vi "Facade.vi"(0 "Data In":T1 caption="数据输入", 2 "Display State In":T4={"method"=enum."None", "current color"=1, "available black position"=[], "available white position"=[], "Interactive Action"=refnum, "row"=0, "column"=0} caption="显示状态输入", 3 "Container State":T7 caption="容器状态") -> (6 "Data Out":T1 caption="数据输出", 7 "Display State Out":T4={"method"=enum."None", "current color"=1, "available black position"=[], "available white position"=[], "Interactive Action"=refnum, "row"=0, "column"=0} caption="显示状态输出", 8 "Action":T3 caption="动作")   [LabVIEW 2011, in "Othello.xctl"]
doc: "查看程序详细说明请访问：http://ruanqizhen.spaces.live.com/blog/cns!5852D4F797C53FB6!3382.entry"
uses:
  Othello.xctl
  Data.ctl
  Control/Pict Ring Chess.ctl
  <vilib>/_xctls/Container State.ctl
  State.ctl
  Control/Method Call.ctl
  Control/Interactive Action.ctl
  <vilib>/_xctls/Action.ctl
  <vilib>/_xctls/XControlSupport.lvlib
panel:
  out "chesses":T1
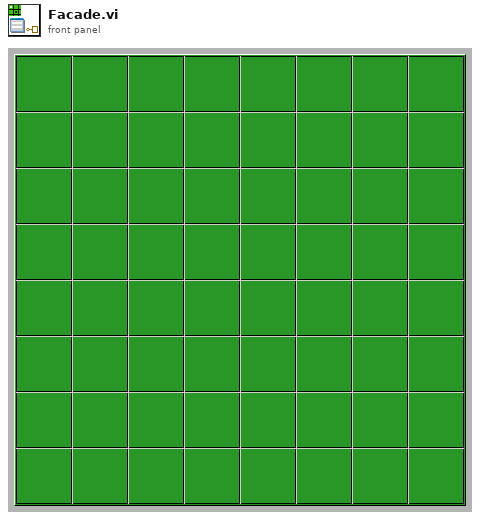
[diagram p1: front panel]
types:
  T1 = typedef "Othello.xctl/Data.ctl" = T2[][]
  T2 = typedef "Othello.xctl/Pict Ring Chess.ctl" = u16
  T3 = typedef "XControlSupport.lvlib/Action.ctl" = cluster{"Data Changed?":bool, "State Changed?":bool, "Action Name":string}
  T4 = typedef "Othello.xctl/State.ctl" = cluster{"method":T5, "current color":T2, "available black position":i32[][], "available white position":i32[][], "Interactive Action":T6, "row":i32, "column":i32}
  T5 = typedef "Othello.xctl/Method Call.ctl" = enum16{"None", "New Game", "Play One"}
  T6 = typedef "Othello.xctl/Interactive Action.ctl" = refnum<user-event>
  T7 = typedef "XControlSupport.lvlib/Container State.ctl" = cluster{"Indicator?":bool, "Run Mode?":bool, " Refnum":refnum<vi>}
  T8 = typedef "LVPoint32TypeDef.ctl" = cluster{"Horizontal":i32, "Vertical":i32}
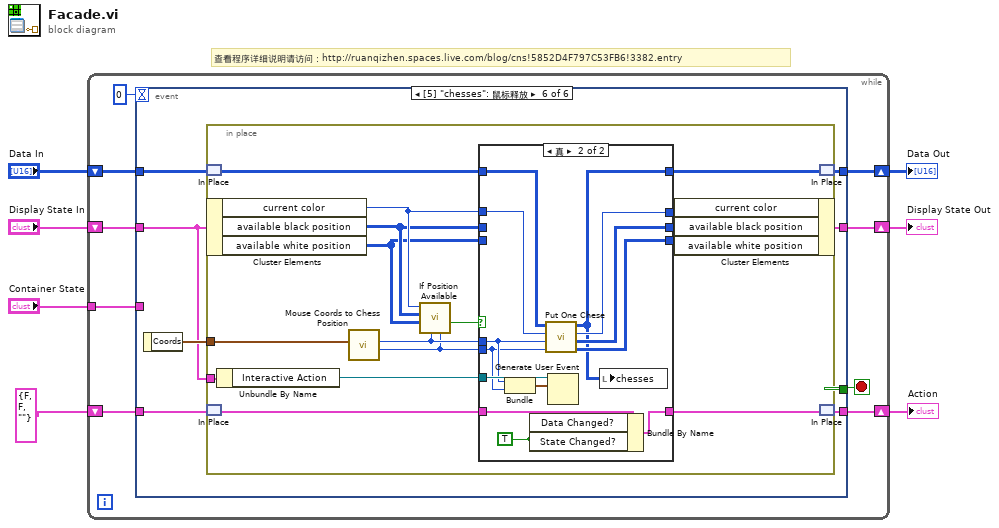
[diagram p0: block diagram]
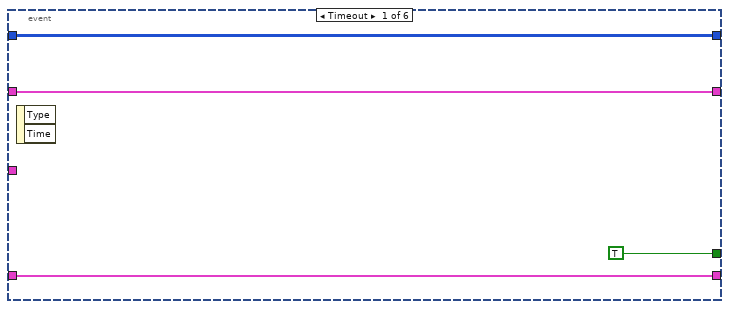
[diagram p2: hidden frame]
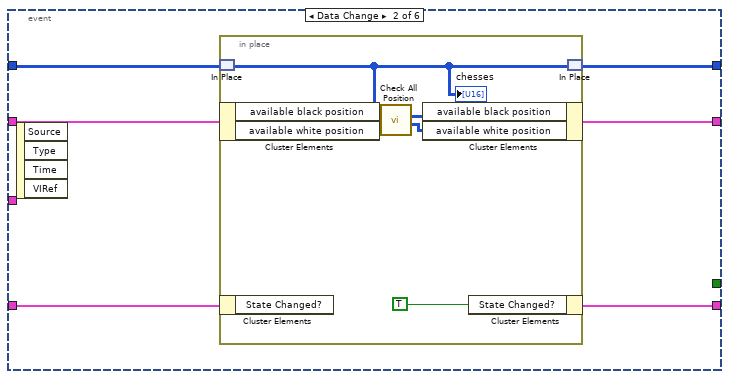
[diagram p3: hidden frame]
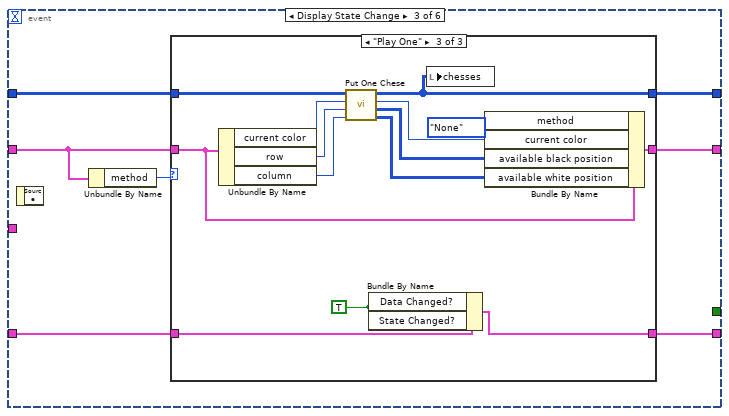
[diagram p4: hidden frame]
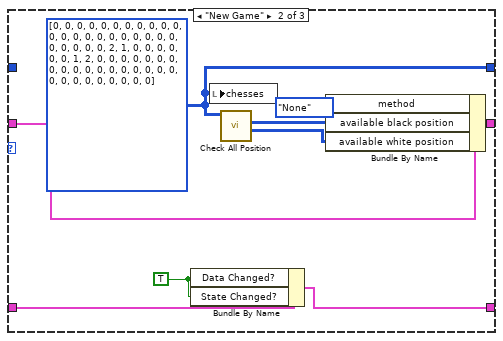
[diagram p6: hidden frame]
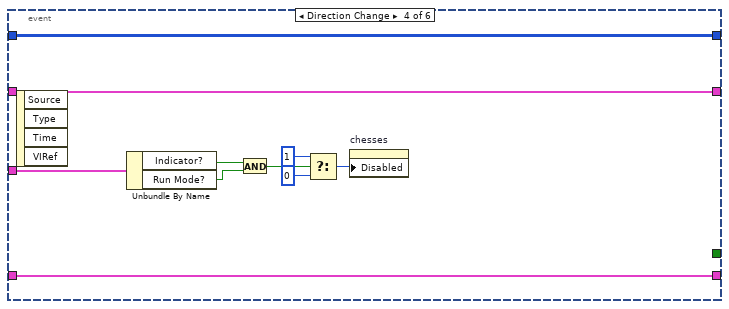
[diagram p7: hidden frame]
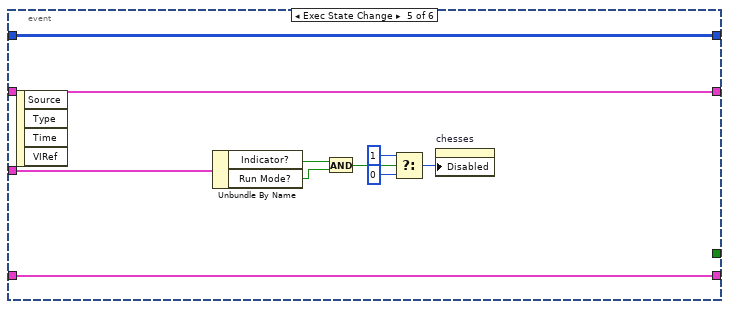
[diagram p8: hidden frame]
diagram:
  # "查看程序详细说明请访问：http://ruanqizhen.spaces.live.com/blog/cns!5852D4F797C53FB6!3382.entry"
  n1 = while {
    shift-right: [w15] -> w4
    shift-left: "Display State In" -> [w16]
    tunnel: "Container State" -> [w12]
    shift-right: [w10] -> w7
    shift-left: "Data In" -> [w11]
    shift-right: [w8] -> w2
    shift-left: T3 {"Data Changed?"=FALSE, "State Changed?"=FALSE, "Action Name"=""} ("Action") -> [w9]
    stop <- w14 stop-if-true
    n2 = event shown="[5] \"chesses\": 鼠标释放" {
      selector: _ -> [_ _ _ _ _ _]
      dyn-events: _ -> [_ _ _ _ _ _]
      timeout: 0 -> [_ _ _ _ _ _]
      tunnel: w16 -> [w18 w25 w33 w72 w83 w86]
      tunnel: [w18 w23 w31 w72 w83 w87] -> w15
      tunnel: [TRUE _ _ _ _ _] -> w14
      tunnel: w12 -> [_ _ _ w73 w74 _]
      tunnel: w11 -> [w17 w22 w36 w71 w82 w89]
      tunnel: [w17 w21 w35 w71 w82 w88] -> w10
      tunnel: [w19 w24 w37 w70 w81 w84] -> w8
      tunnel: w9 -> [w19 w26 w34 w70 w81 w85]
      event Timeout {
        n3 = event-data() -> ()  [unwired: 3 out]
      }
      event Data Change {
        n4 = event-data() -> ()  [unwired: 5 out]
        n5 = in-place {
          n6 = in-place-match #1(w22) -> (w27:T1)
          "chesses" <- w27
          n7 = in-place-cluster #2(w25) -> ()  [unwired: 2 out]
          n8 = in-place-cluster #3(w26) -> ()  [unwired: 1 out]
          n9 = call "Check All Position.vi"("chesses"=w27) -> ("available white position"=w29:i32[][], "available black position"=w28:i32[][])  [unwired: 9 out]
          n10 = in-place-cluster #2("available black position"=w28, "available white position"=w29) -> (w23:T4)
          n11 = in-place-cluster #3("State Changed?"=TRUE ("Data Changed?")) -> (w24:T3)
          n12 = in-place-match #1(w27) -> (w21:T1)
        }
      }
      event Display State Change {
        n13 = event-data() -> ()  [unwired: 2 out]
        n14 = Unbundle By Name(w33) -> ("method"=w32:T5)
        n15 = case shown="\"Play One\"" w32 {
          tunnel: w34 -> [w40 w47 w61]
          tunnel: [w40 w46 w60] -> w37
          tunnel: w36 -> [w39 _ w63]
          tunnel: [w39 w49 w62] -> w35
          tunnel: w33 -> [w38 w41 w55]
          tunnel: [w38 w42 w50] -> w31
          frame "None", Default {
          }
          frame "New Game" {
            w49 = T1 [[0, 0, 0, 0, 0, 0, 0, 0], [0, 0, 0, 0, 0, 0, 0, 0], [0, 0, 0, 0, 0, 0, 0, 0], [0, 0, 0, 2, 1, 0, 0, 0], [0, 0, 0, 1, 2, 0, 0, 0], [0, 0, 0, 0, 0, 0, 0, 0], [0, 0, 0, 0, 0, 0, 0, 0], [0, 0, 0, 0, 0, 0, 0, 0]] ("Data In")
            w48 = TRUE ("Data Changed?")
            n16 = Bundle By Name(cluster=w47, "Data Changed?"=w48, "State Changed?"=w48) -> (w46:T3)
            n17 = local write "chesses"(w49) -> ()
            n18 = call "Check All Position.vi"("chesses"=w49) -> ("available white position"=w44:i32[][], "available black position"=w45:i32[][])  [unwired: 9 out]
            n19 = Bundle By Name(cluster=w41, "method"=Method_Call."None", "available black position"=w45, "available white position"=w44) -> (w42:T4)
          }
          frame "Play One" {
            w59 = TRUE ("Data Changed?")
            n20 = Unbundle By Name(w55) -> ("current color"=w58:T2, "row"=w57:i32, "column"=w56:i32)
            n21 = call "Put One Chese.vi"("column"=w56, "row"=w57, "current color"=w58, "data in"=w63) -> ("available white position"=w51:i32[][], "available black position"=w52:i32[][], "new color"=w53:T2, "data out"=w62:T1)  [unwired: 2 in, 2 out]
            n22 = Bundle By Name(cluster=w61, "Data Changed?"=w59, "State Changed?"=w59) -> (w60:T3)
            n23 = local write "chesses"(w62) -> ()
            n24 = Bundle By Name(cluster=w55, "method"=Method_Call."None", "current color"=w53, "available black position"=w52, "available white position"=w51) -> (w50:T4)
          }
        }
      }
      event Direction Change {
        n25 = event-data() -> ()  [unwired: 5 out]
        n26 = Unbundle By Name(w73) -> ("Indicator?"=w69:bool, "Run Mode?"=w68:bool)
        n27 = And(x=w69, y=w68) -> (x .and. y?=w67:bool)
        n28 = Select(t=u8 1 ("禁用"), s=w67, f=u8 0 ("禁用")) -> (s? t:f=w64:u8)
        n29 = property on="chesses" class="Arr (严格)"("Disabled"=w64) -> ()  [unwired: 2 in, 2 out]
      }
      event Exec State Change {
        n30 = event-data() -> ()  [unwired: 5 out]
        n31 = Unbundle By Name(w74) -> ("Indicator?"=w80:bool, "Run Mode?"=w79:bool)
        n32 = And(x=w80, y=w79) -> (x .and. y?=w78:bool)
        n33 = Select(t=u8 1 ("禁用"), s=w78, f=u8 0 ("禁用")) -> (s? t:f=w75:u8)
        n34 = property on="chesses" class="Arr (严格)"("Disabled"=w75) -> ()  [unwired: 2 in, 2 out]
      }
      event Mouse Up {
        n35 = event-data() -> ("Coords"=w90:T8)  [unwired: 1 out]
        n36 = in-place {
          in-place-border: w90 -> [w106]
          in-place-border: w86 -> [w94]
          n37 = in-place-match #4(w89) -> (w105:T1)
          n38 = in-place-cluster #5(w86) -> ("current color"=w100:T2, "available black position"=w99:i32[][], "available white position"=w98:i32[][])
          n39 = in-place-match #6(w85) -> (w92:T3)
          n40 = Unbundle By Name(w94) -> ("Interactive Action"=w93:T6)
          n41 = call "Mouse Coords to Chess Position.vi"("coords"=w106) -> ("column"=w96:i32, "row"=w97:i32)  [unwired: 9 out]
          n42 = call "If Position Available.vi"("column"=w96, "row"=w97, "available white position"=w98, "available black position"=w99, "current color"=w100) -> ("found?"=w95:bool)  [unwired: 6 out]
          n43 = case shown="真" w95 {
            tunnel: w97 -> [_ w116]
            tunnel: w96 -> [_ w115]
            tunnel: w105 -> [w109 w124]
            tunnel: w100 -> [w108 w123]
            tunnel: [w109 w119] -> w104
            tunnel: [w111 w121] -> w103
            tunnel: [w110 w120] -> w102
            tunnel: w99 -> [w111 _]
            tunnel: w98 -> [w110 _]
            tunnel: [w108 w122] -> w101
            tunnel: w93 -> [_ w118]
            tunnel: w92 -> [w107 w113]
            tunnel: [w107 w112] -> w91
            frame False {
            }
            frame True {
              w114 = TRUE ("Data Changed?")
              n44 = Bundle("row"=w116, "column"=w115) -> (w117:cluster{"row":i32, "column":i32})  [unwired: 1 out]
              n45 = Bundle By Name(cluster=w113, "Data Changed?"=w114, "State Changed?"=w114) -> (w112:T3)
              n46 = call "Put One Chese.vi"("column"=w115, "row"=w116, "current color"=w123, "data in"=w124) -> ("available white position"=w120:i32[][], "available black position"=w121:i32[][], "new color"=w122:T2, "data out"=w119:T1)  [unwired: 2 in, 2 out]
              n47 = Generate User Event(user event=w118, event data cluster=w117) -> ()  [unwired: 1 in, 2 out]
              n48 = local write "chesses"(w119) -> ()
            }
          }
          n49 = in-place-cluster #5("current color"=w101, "available black position"=w103, "available white position"=w102) -> (w87:T4)
          n50 = in-place-match #4(w104) -> (w88:T1)
          n51 = in-place-match #6(w91) -> (w84:T3)
        }
      }
    }
  }
  "Display State Out" <- w4
  "Data Out" <- w7
  "Action" <- w2
